vi "LSX Set Motor Table Patch.vi"(8 "error in (no error)":errorcluster, 10 "bActive":i32, 11 "lLSID":i32) -> (0 "error out":errorcluster, 3 "function return":i32)   [LabVIEW 2018, in "Tango.lvlib"]
doc: "TANGOAPI int TANGOCALL LSX_SetMotorTablePatch (int lLSID, BOOL bActive);"
uses:
  Tango.lvlib
  SubVIs/Tango_DLL.dll
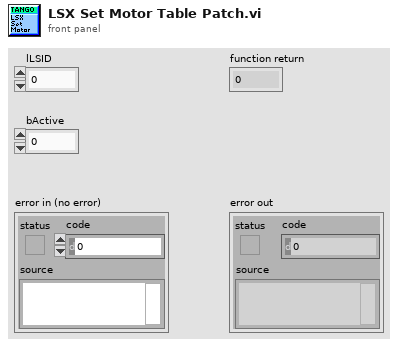
[diagram p1: front panel]
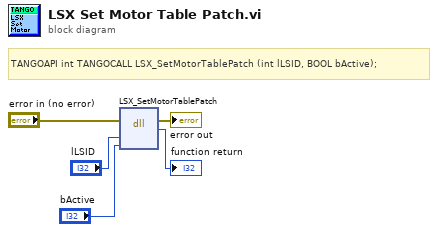
[diagram p0: block diagram]
diagram:
  # "TANGOAPI int TANGOCALL LSX_SetMotorTablePatch (int lLSID, BOOL bActive);"
  n1 = dll-call lib="C:/Users/Familie/Documents/LabviewIX81/lib/TANGO Stage/SubVIs/Tango_DLL.*" fn="LSX_SetMotorTablePatch"(error in="error in (no error)", "lLSID"="lLSID", "bActive"="bActive") -> (error out=→"error out":errorcluster, →"function return":i32)  [unwired: 4 in, 1 out]
